vi "Admin.vi"() -> ()   [LabVIEW 2017]
panel:
  out "array":string[][](array[string])
  out "Tab Control":enum32{"Login", "Admin", "Usuario", "ADMIN"}(tab)
  in  "Ingresar":bool
  in  "Contraseña":string
  in  "Usuario":string
  in  "AddContraseña":string
  in  "addUsuario":string
  in  "Agregar":bool
  out "Sesion Iniciada Por:":string
  in  "Volver":bool
  in  "Lista":bool
  out "String":string
  in  "BORRAR":bool
  in  "Ingrese el usuario que desea eliminar":string
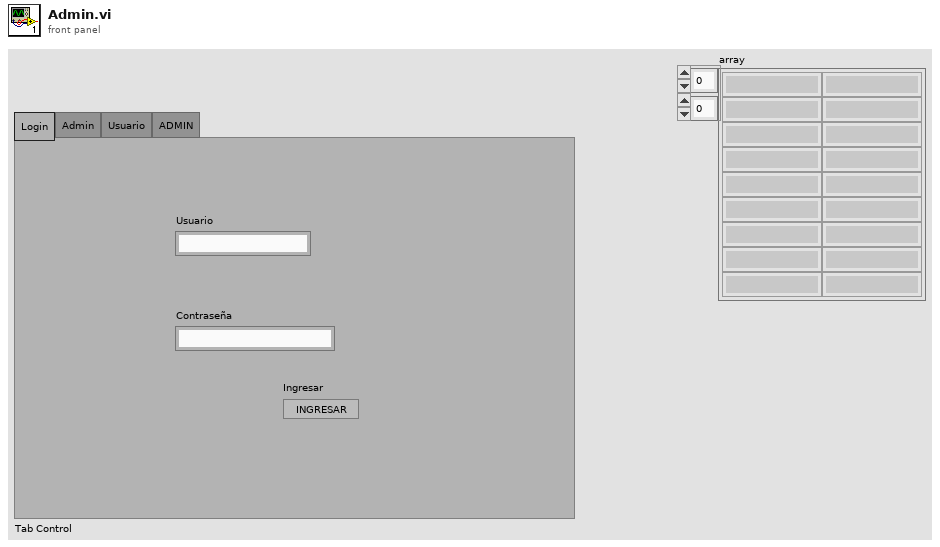
[diagram p1: front panel]
types:
  T1 = enum16{"open", "replace", "create", "open or create", "replace or create", "replace or create with confirmation"}
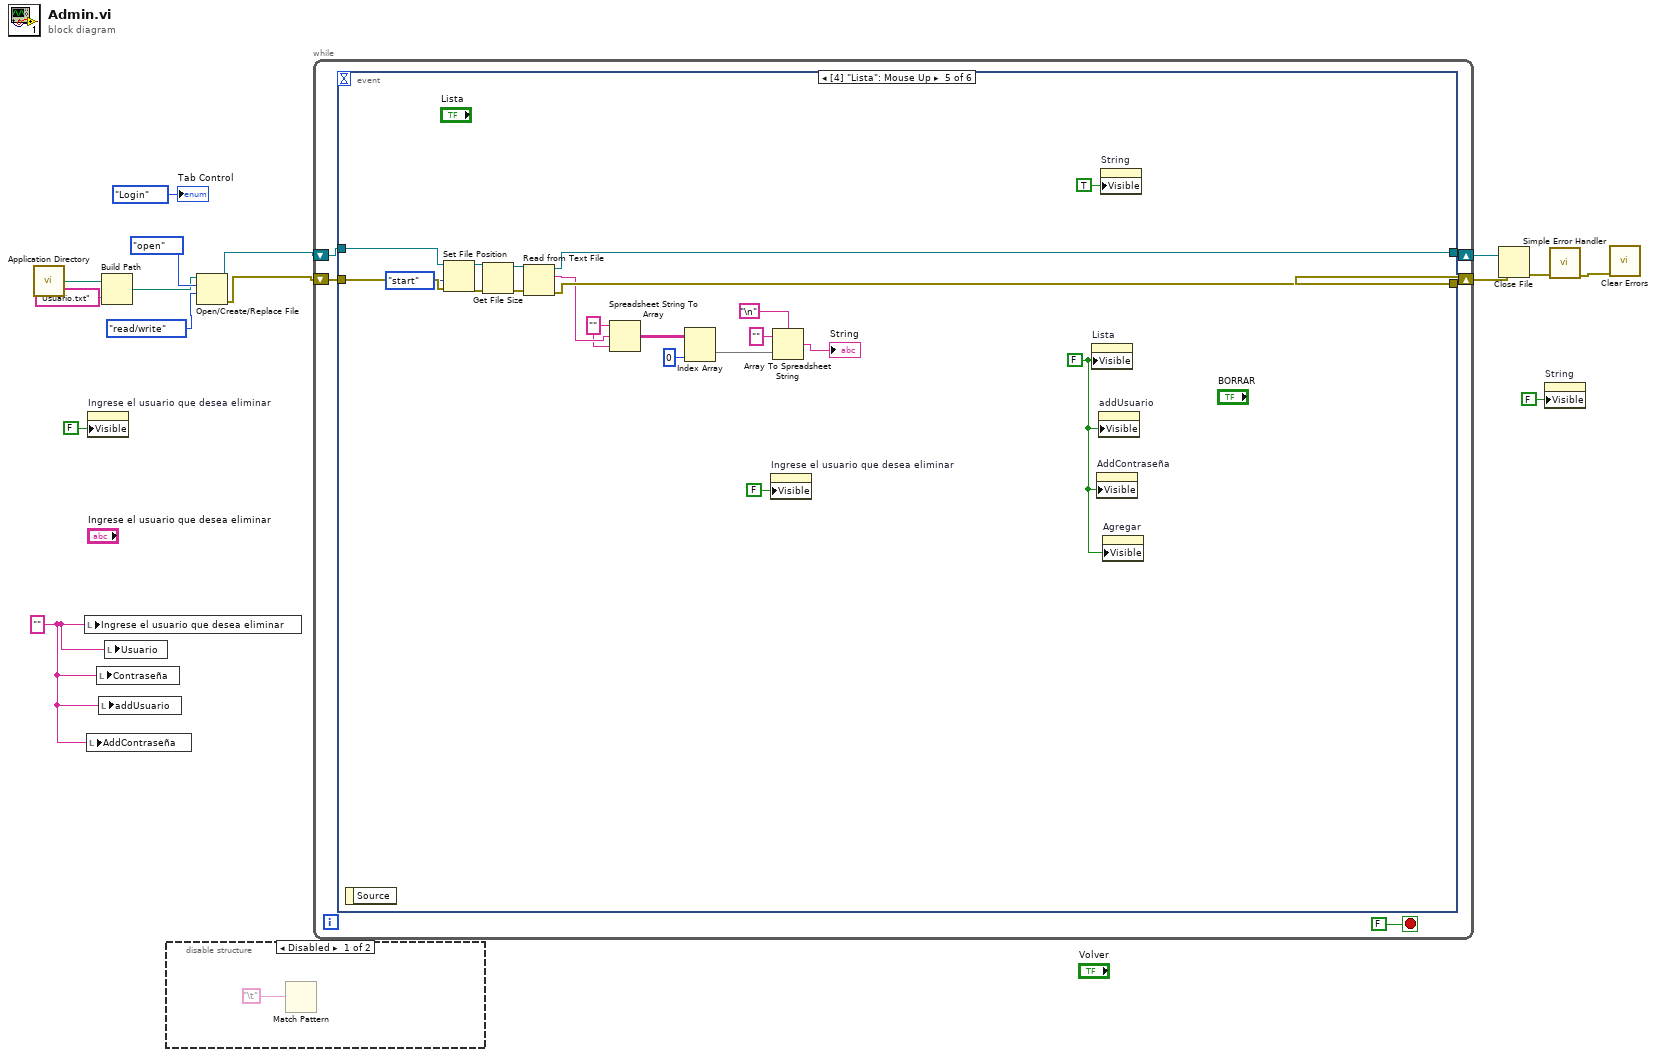
[diagram p0: block diagram]
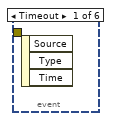
[diagram p3: hidden frame]
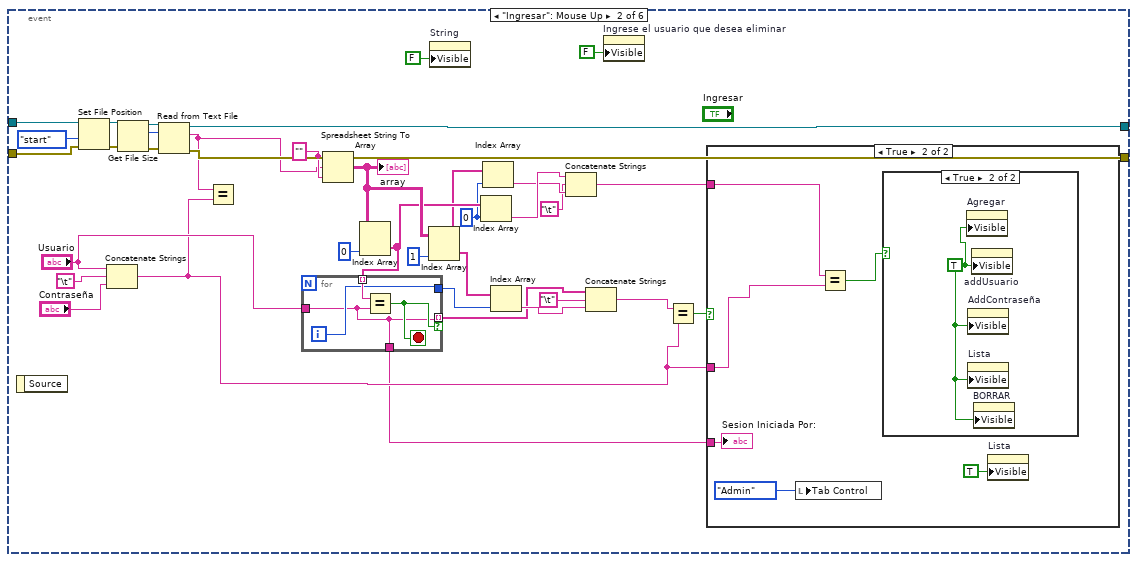
[diagram p4: hidden frame]
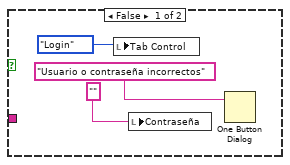
[diagram p5: hidden frame]
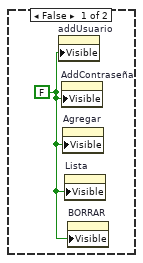
[diagram p6: hidden frame]
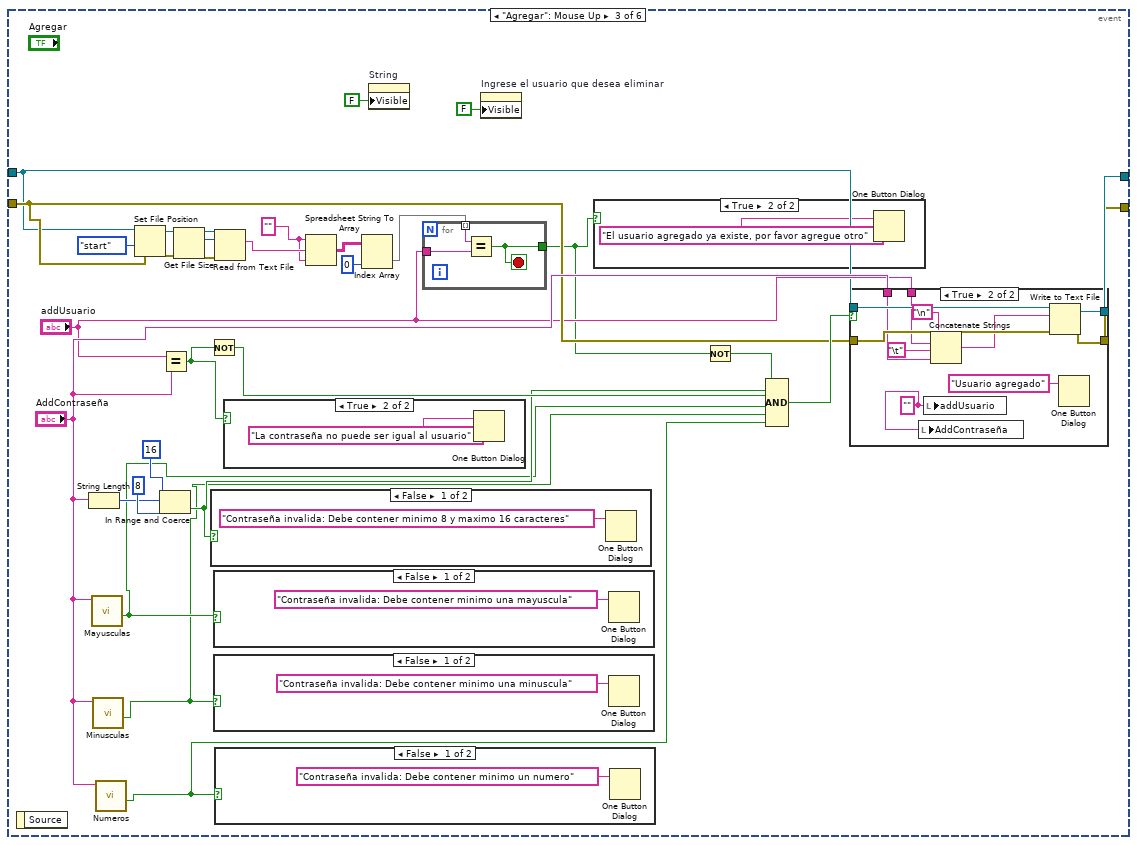
[diagram p7: hidden frame]
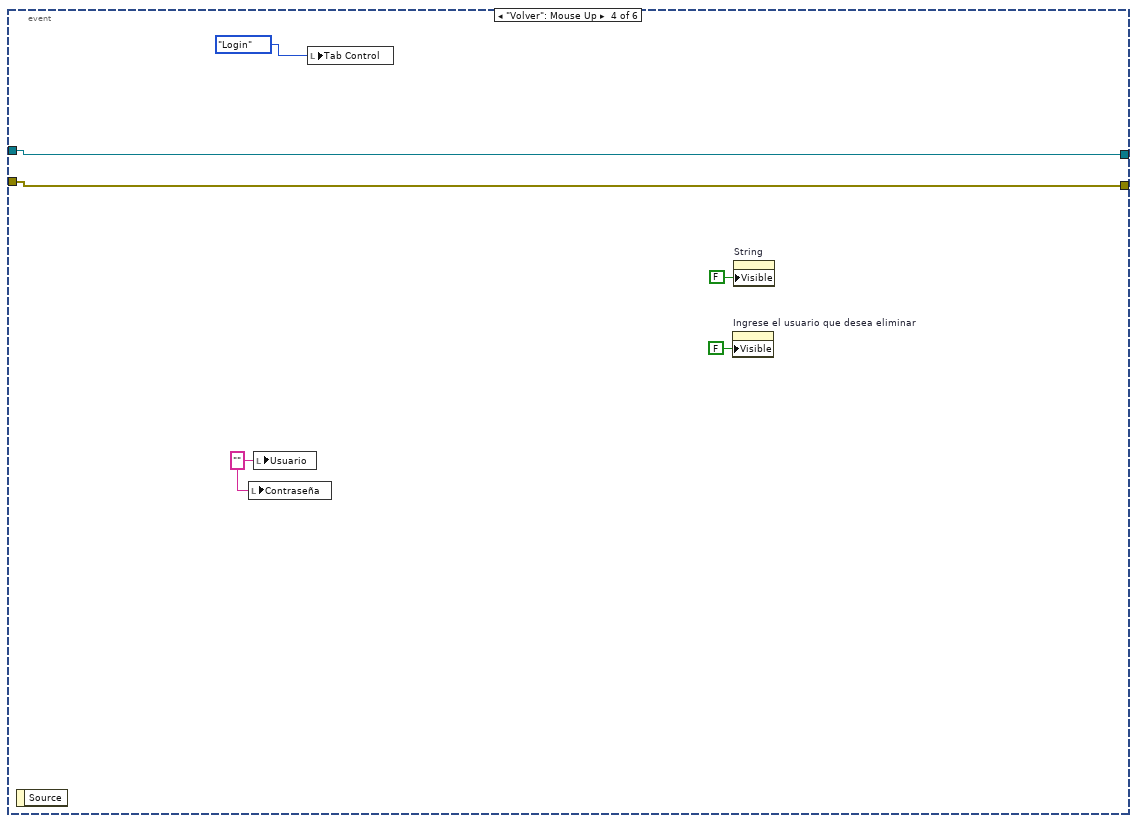
[diagram p15: hidden frame]
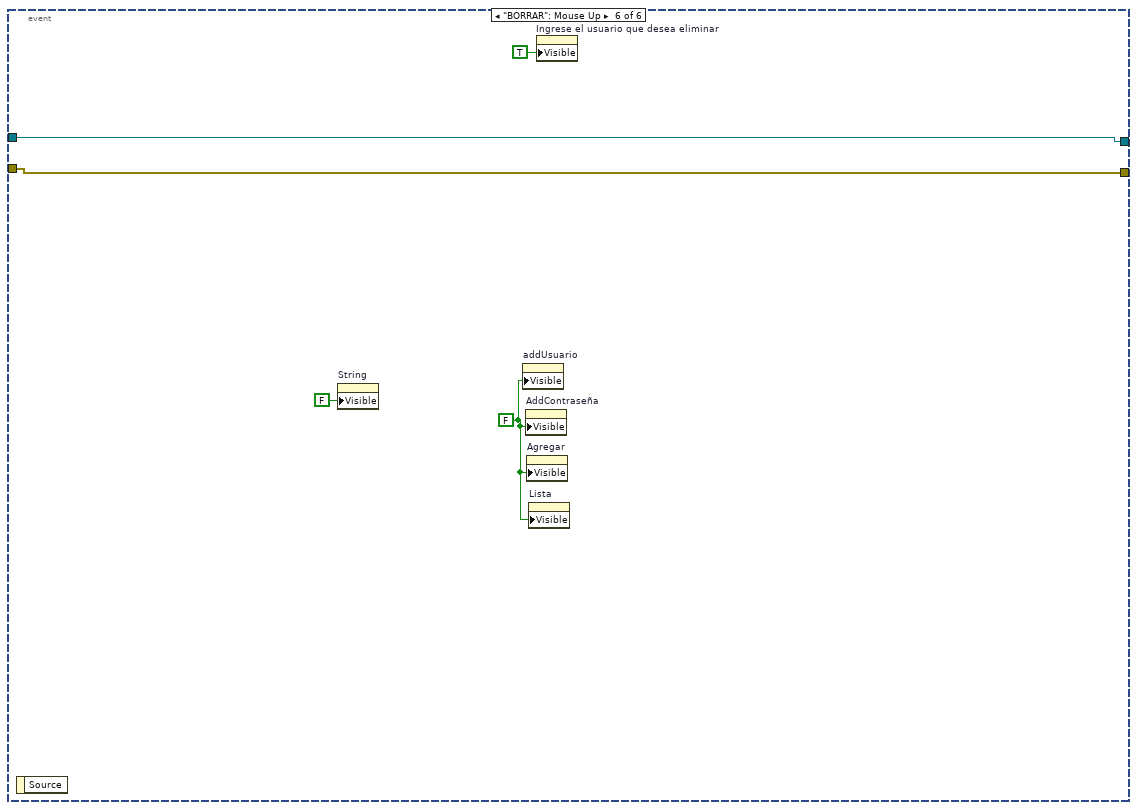
[diagram p16: hidden frame]
diagram:
  w1 = "" ("Usuario")
  n1 = call <vilib>:"Application Directory.vi"() -> ("Application Directory"=w15:path)
  n2 = local write "Ingrese el usuario que desea eliminar"(w1) -> ()
  n3 = local write "AddContraseña"(w1) -> ()
  n4 = property on="Ingrese el usuario que desea eliminar" class="Str"("Visible"=FALSE) -> ()  [unwired: 2 in, 2 out]
  n5 = local write "Contraseña"(w1) -> ()
  n6 = local write "addUsuario"(w1) -> ()
  n7 = Build Path(base path=w15, name or relative path="Usuario.txt") -> (appended path=w11:path)
  n8 = local write "Usuario"(w1) -> ()
  n9 = disable-structure shown="Disabled" {
    frame Disabled {
      n10 = Match Pattern(regular expression="\t") -> (match substring=w16:string)  [unwired: 2 in, 3 out]
    }
    frame Enabled {
    }
  }
  n11 = Open/Create/Replace File(file path (use dialog)=w11, operation (0:open)=T1."open", access (0:read/write)=enum16{"read/write", "read-only", "write-only"}."read/write") -> (refnum out=w6:refnum<file>, error out=w5:errorcluster)  [unwired: 3 in, 1 out]
  n12 = while {
    shift-right: [w19] -> w8
    shift-left: w6 -> [w21]
    shift-right: [w18] -> w7
    shift-left: w5 -> [w20]
    stop <- FALSE stop-if-true
    n13 = event shown="[4] \"Lista\": Mouse Up" {
      selector: _ -> [_ _ _ _ _ _]
      dyn-events: _ -> [_ _ _ _ _ _]
      timeout: _ -> [_ _ _ _ _ _]
      tunnel: w21 -> [_ w57 w77 w129 w149 w154]
      tunnel: w20 -> [_ w55 w89 w128 w146 w153]
      tunnel: [_ w49 w103 w129 w144 w154] -> w19
      tunnel: [_ w48 w102 w128 w143 w153] -> w18
      event Timeout {
        n14 = event-data() -> ()  [unwired: 1 in, 3 out]
      }
      event "Ingresar": Mouse Up {
        w32 = 0 ("index")
        w46 = "" ("format string")
        n15 = event-data() -> ()  [unwired: 1 in, 1 out]
        n16 = Set File Position(refnum=w57, from (0:start)=enum16{"start", "end", "current"}."start", error in=w55) -> (refnum out=w53:refnum<file>, error out=w54:errorcluster)  [unwired: 1 in]
        n17 = Concatenate Strings("Usuario", "\t", "Contraseña") -> (w34:string)
        n18 = Get File Size(file=w53, error in=w54) -> (refnum out=w52:refnum<file>, size (in bytes)=w51:i64, 0:w50:errorcluster)
        n19 = Read from Text File(file (use dialog)=w52, count=w51, error in=w50) -> (refnum out=w49:refnum<file>, text=w39:string, error out=w48:errorcluster)  [unwired: 1 in, 1 out]
        n20 = Equal?(x=w39, y=w34) -> ()  [unwired: 1 out]
        n21 = Spreadsheet String To Array(format string=w46, spreadsheet string=w39, array type (2D Dbl)=w46) -> (array=w35:string[][])  [unwired: 1 in]
        "array" <- w35
        n22 = Index Array(array=w35, index (col)=0 ("disabled index (col)")) -> (element=w33:string[])  [unwired: 1 in]
        n23 = for {
          tunnel: w33 -> [w61] mode=indexing
          tunnel: "Usuario" -> [w58]
          tunnel: [w58] -> w26 mode=indexing if=w60
          tunnel: [w59] -> w37
          tunnel: [w58] -> w25
          i -> [w59]
          stop <- w60 stop-if-true
          n24 = Equal?(x=w61, y=w58) -> (x = y?=w60:bool)
        }
        n25 = Index Array(array=w35, index (col)=1 ("disabled index (col)")) -> (element=w27:string[])  [unwired: 1 in]
        n26 = property on="String" class="Str"("Visible"=FALSE) -> ()  [unwired: 2 in, 2 out]
        n27 = Index Array(array=w33, index=w32) -> (element=w31:string)
        n28 = Index Array(array=w27, index=w32) -> (element=w30:string)
        n29 = Index Array(array=w27, index=w37) -> (element=w36:string)
        n30 = Concatenate Strings(w31, "\t", w30) -> (w28:string)
        n31 = Concatenate Strings(w26, "\t", w36) -> (w41:string)
        n32 = property on="Ingrese el usuario que desea eliminar" class="Str"("Visible"=FALSE) -> ()  [unwired: 2 in, 2 out]
        n33 = Equal?(x=w41, y=w34) -> (x = y?=w40:bool)
        n34 = case shown="True" w40 {
          tunnel: w34 -> [_ w69]
          tunnel: w28 -> [_ w68]
          tunnel: w25 -> [_ w66]
          frame False {
            n35 = local write "Tab Control"(enum32{"Login", "Admin", "Usuario", "ADMIN"}."Login" ("Tab Control")) -> ()
            n36 = local write "Contraseña"("" ("Usuario")) -> ()
            n37 = One Button Dialog(message="Usuario o contraseña incorrectos") -> ()  [unwired: 1 in, 1 out]
          }
          frame True {
            n38 = local write "Tab Control"(enum32{"Login", "Admin", "Usuario", "ADMIN"}."Admin" ("Tab Control")) -> ()
            n39 = Equal?(x=w68, y=w69) -> (x = y?=w67:bool)
            n40 = case shown="True" w67 {
              frame False {
                w71 = FALSE ("Visible")
                n41 = property on="addUsuario" class="Str"("Visible"=w71) -> ()  [unwired: 2 in, 2 out]
                n42 = property on="AddContraseña" class="Str"("Visible"=w71) -> ()  [unwired: 2 in, 2 out]
                n43 = property on="Agregar" class="Bool (strict)"("Visible"=w71) -> ()  [unwired: 2 in, 2 out]
                n44 = property on="Lista" class="Bool (strict)"("Visible"=w71) -> ()  [unwired: 2 in, 2 out]
                n45 = property on="BORRAR" class="Bool (strict)"("Visible"=w71) -> ()  [unwired: 2 in, 2 out]
              }
              frame True {
                w72 = TRUE ("Visible")
                n46 = property on="Agregar" class="Bool (strict)"("Visible"=w72) -> ()  [unwired: 2 in, 2 out]
                n47 = property on="AddContraseña" class="Str"("Visible"=w72) -> ()  [unwired: 2 in, 2 out]
                n48 = property on="Lista" class="Bool (strict)"("Visible"=w72) -> ()  [unwired: 2 in, 2 out]
                n49 = property on="addUsuario" class="Str"("Visible"=w72) -> ()  [unwired: 2 in, 2 out]
                n50 = property on="BORRAR" class="Bool (strict)"("Visible"=w72) -> ()  [unwired: 2 in, 2 out]
              }
            }
            n51 = property on="Lista" class="Bool (strict)"("Visible"=TRUE) -> ()  [unwired: 2 in, 2 out]
            "Sesion Iniciada Por:" <- w66
          }
        }
      }
      event "Agregar": Mouse Up {
        w82 = "" ("format string")
        n52 = event-data() -> ()  [unwired: 1 in, 1 out]
        n53 = String Length(string="AddContraseña") -> (length=w99:i32)
        n54 = call "Mayusculas.vi"("Palabra"="AddContraseña") -> ("Boolean"=w94:bool)  [unwired: 8 in, 2 out]
        n55 = call "Minusculas.vi"("Palabra"="AddContraseña") -> ("Boolean"=w93:bool)  [unwired: 8 in, 2 out]
        n56 = call "Numeros.vi"("Palabra"="AddContraseña") -> ("Boolean"=w92:bool)  [unwired: 8 in, 2 out]
        n57 = Set File Position(refnum=w77, from (0:start)=enum16{"start", "end", "current"}."start", error in=w89) -> (refnum out=w85:refnum<file>, error out=w88:errorcluster)  [unwired: 1 in]
        n58 = In Range and Coerce(upper limit=16, x=w99, lower limit=8) -> (In Range?=w95:bool)  [unwired: 1 out]
        n59 = Equal?(x="addUsuario", y="AddContraseña") -> (x = y?=w98:bool)
        n60 = Get File Size(file=w85, error in=w88) -> (refnum out=w86:refnum<file>, size (in bytes)=w90:i64, 0:w87:errorcluster)
        n61 = Not(x=w98) -> (.not. x?=w96:bool)
        n62 = case shown="False" w95 {
          frame False {
            n63 = One Button Dialog(message="Contraseña invalida: Debe contener minimo 8 y maximo 16 caracteres") -> ()  [unwired: 1 in, 1 out]
          }
          frame True {
          }
        }
        n64 = case shown="False" w94 {
          frame False {
            n65 = One Button Dialog(message="Contraseña invalida: Debe contener minimo una mayuscula") -> ()  [unwired: 1 in, 1 out]
          }
          frame True {
          }
        }
        n66 = case shown="False" w93 {
          frame False {
            n67 = One Button Dialog(message="Contraseña invalida: Debe contener minimo una minuscula") -> ()  [unwired: 1 in, 1 out]
          }
          frame True {
          }
        }
        n68 = Read from Text File(file (use dialog)=w86, count=w90, error in=w87) -> (text=w83:string)  [unwired: 1 in, 3 out]
        n69 = case shown="False" w92 {
          frame False {
            n70 = One Button Dialog(message="Contraseña invalida: Debe contener minimo un numero") -> ()  [unwired: 1 in, 1 out]
          }
          frame True {
          }
        }
        n71 = case shown="True" w98 {
          frame False {
          }
          frame True {
            n72 = One Button Dialog(message="La contraseña no puede ser igual al usuario") -> ()  [unwired: 1 in, 1 out]
          }
        }
        n73 = Spreadsheet String To Array(format string=w82, spreadsheet string=w83, array type (2D Dbl)=w82) -> (array=w80:string[][])  [unwired: 1 in]
        n74 = Index Array(array=w80, index (col)=0 ("disabled index (col)")) -> (element=w78:string[])  [unwired: 1 in]
        n75 = property on="String" class="Str"("Visible"=FALSE) -> ()  [unwired: 2 in, 2 out]
        n76 = for {
          tunnel: "addUsuario" -> [w107]
          tunnel: w78 -> [w106] mode=indexing
          tunnel: [w105] -> w76
          stop <- w105 stop-if-true
          n77 = Equal?(x=w106, y=w107) -> (x = y?=w105:bool)
        }
        n78 = property on="Ingrese el usuario que desea eliminar" class="Str"("Visible"=FALSE) -> ()  [unwired: 2 in, 2 out]
        n79 = case shown="True" w76 {
          frame False {
          }
          frame True {
            n80 = One Button Dialog(message="El usuario agregado ya existe, por favor agregue otro") -> ()  [unwired: 1 in, 1 out]
          }
        }
        n81 = Not(x=w76) -> (.not. x?=w75:bool)
        n82 = Compound Arithmetic op=AND(w75, w95, w96, w94, w93, w92) -> (w91:bool)
        n83 = case shown="True" w91 {
          tunnel: w77 -> [w112 w123]
          tunnel: w89 -> [w111 w122]
          tunnel: [w112 w121] -> w103
          tunnel: [w111 w120] -> w102
          tunnel: "addUsuario" -> [_ w119]
          tunnel: "AddContraseña" -> [_ w118]
          frame False {
          }
          frame True {
            w113 = "" ("addUsuario")
            n84 = local write "AddContraseña"(w113) -> ()
            n85 = local write "addUsuario"(w113) -> ()
            n86 = Concatenate Strings("\n", w119, "\t", w118) -> (w117:string)
            n87 = Write to Text File(file (use dialog)=w123, text=w117, error in=w122) -> (refnum out=w121:refnum<file>, error out=w120:errorcluster)  [unwired: 1 in, 1 out]
            n88 = One Button Dialog(message="Usuario agregado") -> ()  [unwired: 1 in, 1 out]
          }
        }
      }
      event "Volver": Mouse Up {
        w130 = "" ("Usuario")
        n89 = event-data() -> ()  [unwired: 1 in, 1 out]
        n90 = local write "Contraseña"(w130) -> ()
        n91 = local write "Usuario"(w130) -> ()
        n92 = local write "Tab Control"(enum32{"Login", "Admin", "Usuario", "ADMIN"}."Login" ("Tab Control")) -> ()
        n93 = property on="Ingrese el usuario que desea eliminar" class="Str"("Visible"=FALSE) -> ()  [unwired: 2 in, 2 out]
        n94 = property on="String" class="Str"("Visible"=FALSE) -> ()  [unwired: 2 in, 2 out]
      }
      event "Lista": Mouse Up {
        w133 = FALSE ("Visible")
        w141 = "" ("format string")
        n95 = event-data() -> ()  [unwired: 1 in, 1 out]
        n96 = Set File Position(refnum=w149, from (0:start)=enum16{"start", "end", "current"}."start", error in=w146) -> (refnum out=w151:refnum<file>, error out=w147:errorcluster)  [unwired: 1 in]
        n97 = Get File Size(file=w151, error in=w147) -> (refnum out=w150:refnum<file>, 0:w148:errorcluster)  [unwired: 1 out]
        n98 = Read from Text File(file (use dialog)=w150, error in=w148) -> (refnum out=w144:refnum<file>, text=w142:string, error out=w143:errorcluster)  [unwired: 2 in, 1 out]
        n99 = Spreadsheet String To Array(format string=w141, spreadsheet string=w142, array type (2D Dbl)=w141) -> (array=w140:string[][])  [unwired: 1 in]
        n100 = Index Array(array=w140, index (col)=0 ("disabled index (col)")) -> (element=w137:string[])  [unwired: 1 in]
        n101 = property on="Ingrese el usuario que desea eliminar" class="Str"("Visible"=FALSE) -> ()  [unwired: 2 in, 2 out]
        n102 = Array To Spreadsheet String(delimiter (Tab)="\n", array=w137, 3:"" ("format string")) -> (spreadsheet string=→"String":string)
        n103 = property on="Lista" class="Bool (strict)"("Visible"=w133) -> ()  [unwired: 2 in, 2 out]
        n104 = property on="AddContraseña" class="Str"("Visible"=w133) -> ()  [unwired: 2 in, 2 out]
        n105 = property on="addUsuario" class="Str"("Visible"=w133) -> ()  [unwired: 2 in, 2 out]
        n106 = property on="String" class="Str"("Visible"=TRUE) -> ()  [unwired: 2 in, 2 out]
        n107 = property on="Agregar" class="Bool (strict)"("Visible"=w133) -> ()  [unwired: 2 in, 2 out]
      }
      event "BORRAR": Mouse Up {
        w156 = FALSE ("Visible")
        n108 = event-data() -> ()  [unwired: 1 in, 1 out]
        n109 = property on="String" class="Str"("Visible"=FALSE) -> ()  [unwired: 2 in, 2 out]
        n110 = property on="addUsuario" class="Str"("Visible"=w156) -> ()  [unwired: 2 in, 2 out]
        n111 = property on="AddContraseña" class="Str"("Visible"=w156) -> ()  [unwired: 2 in, 2 out]
        n112 = property on="Agregar" class="Bool (strict)"("Visible"=w156) -> ()  [unwired: 2 in, 2 out]
        n113 = property on="Lista" class="Bool (strict)"("Visible"=w156) -> ()  [unwired: 2 in, 2 out]
        n114 = property on="Ingrese el usuario que desea eliminar" class="Str"("Visible"=TRUE) -> ()  [unwired: 2 in, 2 out]
      }
    }
  }
  n115 = Close File(refnum=w8, error in=w7) -> (error out=w9:errorcluster)  [unwired: 1 out]
  n116 = property on="String" class="Str"("Visible"=FALSE) -> ()  [unwired: 2 in, 2 out]
  n117 = call <vilib>:"Simple Error Handler.vi"("error in (no error)"=w9) -> ("error out"=w10:errorcluster)  [unwired: 4 in, 4 out]
  n118 = call <vilib>:"Clear Errors.vi"("error in (no error)"=w10) -> ()  [unwired: 5 in, 2 out]
  "Tab Control" <- enum32{"Login", "Admin", "Usuario", "ADMIN"}."Login" ("Tab Control")
